vi "Remove Port HW Entry.vi"(6 "InstrumentHandle_port":u32, 9 "portId":u32, 10 "boardId":u32, 11 "hw_data in":T1) -> (3 "hw_data out":T1)   [LabVIEW 2020, in "AIM664LV.lvlib"]
uses:
  AIM664LV.lvlib
  _controls/hwEntry_data.ctl
  _controls/hwEntryBoardHandleMap.ctl
  _controls/hwEntryBoardResource.ctl
  _controls/hwEntryPortResource.ctl
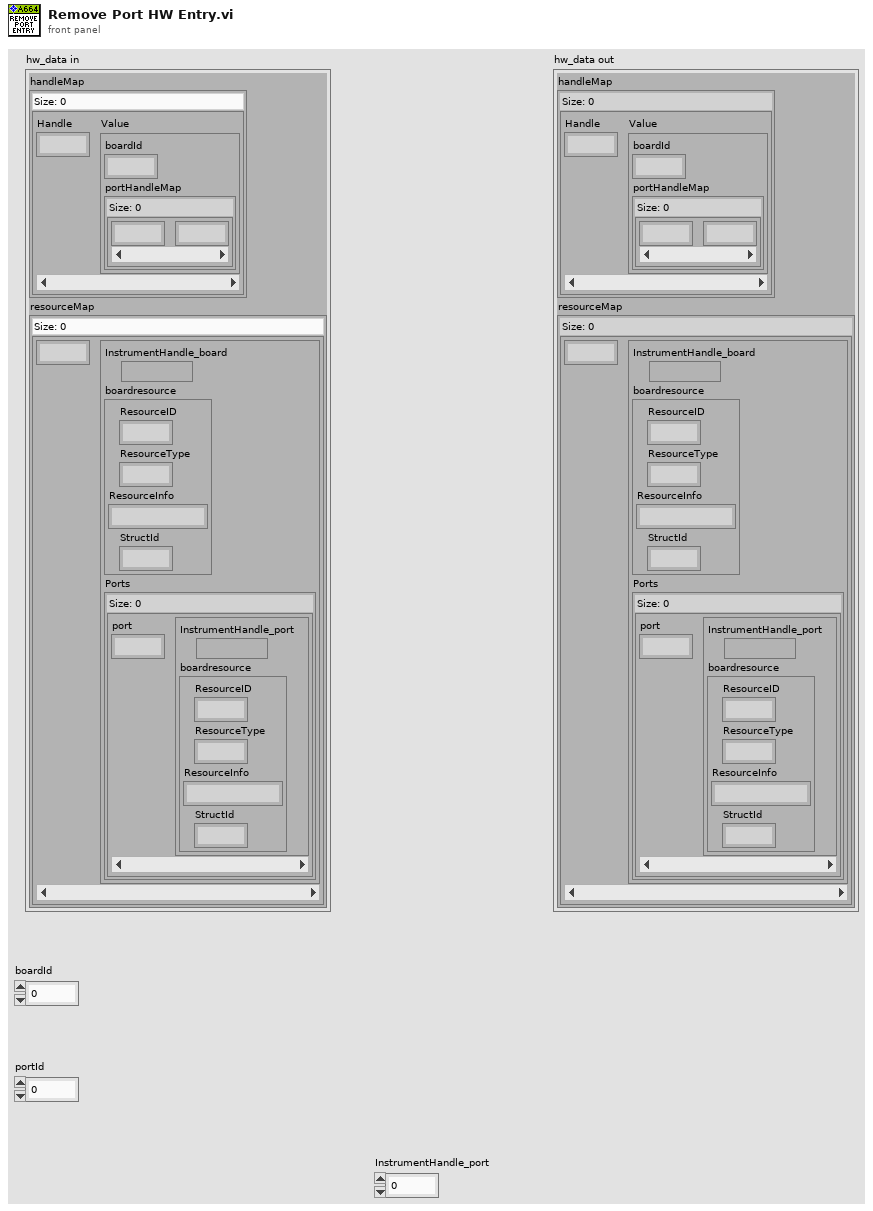
[diagram p1: front panel]
types:
  T1 = typedef "AIM664LV.lvlib/hwEntry_data.ctl" = cluster{"handleMap":map{u32, T2}, "resourceMap":map{u32, T3}}
  T2 = typedef "AIM664LV.lvlib/hwEntryBoardHandleMap.ctl" = cluster{"boardId":u32, "portHandleMap":map{u32, u32}}
  T3 = typedef "AIM664LV.lvlib/hwEntryBoardResource.ctl" = cluster{"InstrumentHandle_board":u32, "boardresource":cluster{"ResourceID":u32, "ResourceType":u32, "ResourceInfo":string, "StructId":u32}, "Ports":map{u32, T4}}
  T4 = typedef "AIM664LV.lvlib/hwEntryPortResource.ctl" = cluster{"InstrumentHandle_port":u32, "boardresource":cluster{"ResourceID":u32, "ResourceType":u32, "ResourceInfo":string, "StructId":u32}}
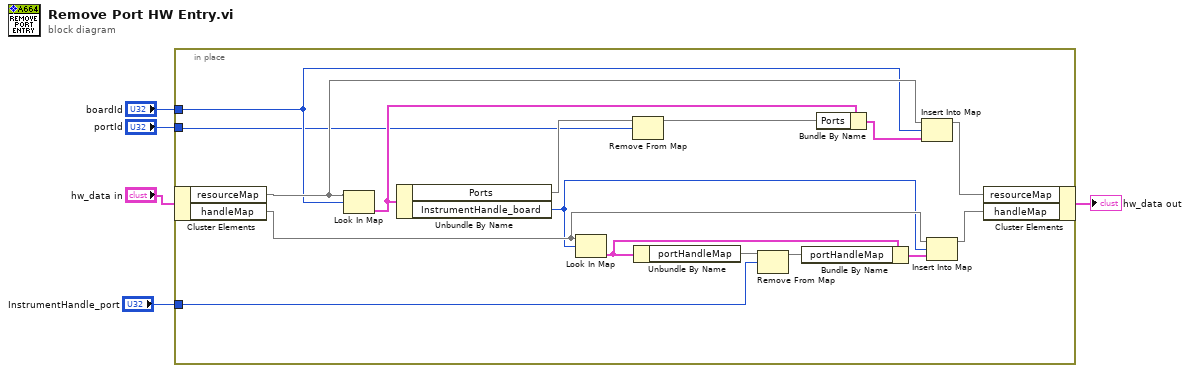
[diagram p0: block diagram]
diagram:
  n1 = in-place {
    in-place-border: "boardId" -> [w9]
    in-place-border: "InstrumentHandle_port" -> [w15]
    in-place-border: "portId" -> [w6]
    n2 = in-place-cluster #1("hw_data in") -> ("resourceMap"=w11:map{u32, T3}, "handleMap"=w20:map{u32, T2})
    n3 = Look In Map(map=w11, key=w9) -> (value=w13:T3)  [unwired: 1 in, 1 out]
    n4 = Unbundle By Name(w13) -> ("Ports"=w14:map{u32, T4}, "InstrumentHandle_board"=w17:u32)
    n5 = Look In Map(map=w20, key=w17) -> (value=w19:T2)  [unwired: 1 in, 1 out]
    n6 = Remove From Map(10:w6, 11:w14) -> (3:w12:map{u32, T4})  [unwired: 2 out]
    n7 = Unbundle By Name(w19) -> ("portHandleMap"=w21:map{u32, u32})
    n8 = Remove From Map(10:w15, 11:w21) -> (3:w16:map{u32, u32})  [unwired: 2 out]
    n9 = Bundle By Name(cluster=w19, "portHandleMap"=w16) -> (w18:T2)
    n10 = Bundle By Name(cluster=w13, "Ports"=w12) -> (w10:T3)
    n11 = Insert Into Map(map in=w11, key=w9, value=w10) -> (map out=w8:map{u32, T3})  [unwired: 2 out]
    n12 = Insert Into Map(map in=w20, key=w17, value=w18) -> (map out=w7:map{u32, T2})  [unwired: 2 out]
    n13 = in-place-cluster #1("resourceMap"=w8, "handleMap"=w7) -> (→"hw_data out":T1)
  }
